vi "Get Sniffer Callbacks.vi"(8 "error in (no error)":errorcluster, 11 "Endpoint in":refnum<class "Endpoint.lvclass">) -> (0 "error out":errorcluster, 2 "Sniffer Callbacks":T1[](array[typedef]), 3 "Endpoint out":refnum<class "Endpoint.lvclass">)   [LabVIEW 2020, in "Stream.lvlib" / "Endpoint.lvclass"]
uses:
  Endpoint.lvclass
  State Callback.ctl
  Endpoint.lvclass/Endpoint.ctl
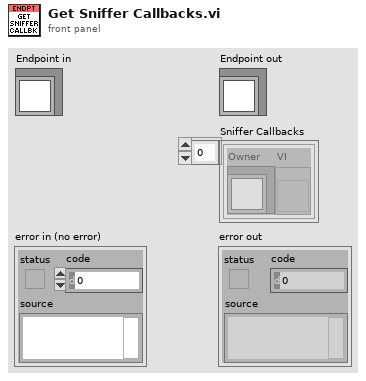
[diagram p1: front panel]
types:
  T1 = typedef "Stream.lvlib/Endpoint.lvclass/State Callback.ctl" = cluster{"Owner":refnum<class>, "VI":refnum<vi>}
  T2 = typedef "Stream.lvlib/Endpoint.lvclass/Ref Data.ctl" = cluster{"URI":refnum<class "URI.lvclass">, "State Callbacks":T1[], "Open":bool, "Mode":T3, "Sniffer Callbacks":T1[]}
  T3 = typedef "Stream.lvlib/Mode.ctl" = enum16{"Raw", "Buffered", "LineTerm", "Message"}
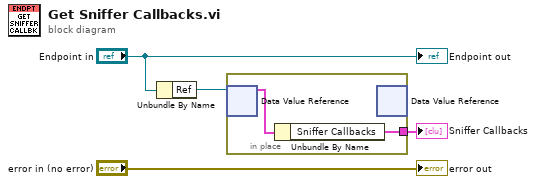
[diagram p0: block diagram]
diagram:
  n1 = Unbundle By Name("Endpoint in") -> ("Ref"=w3:refnum<data-value>)
  n2 = in-place {
    in-place-border: [w5] -> w1
    n3 = in-place-dvr #1(w3) -> (w6:T2)  [unwired: 1 out]
    n4 = Unbundle By Name(w6) -> ("Sniffer Callbacks"=w5:T1[])
    n5 = in-place-dvr #1() -> ()  [unwired: 1 in, 2 out]
  }
  "Sniffer Callbacks" <- w1
  "error out" <- "error in (no error)"
  "Endpoint out" <- "Endpoint in"
